vi "Translate Percent Codes.vi"(11 "String":string) -> (3 "String 2":string)   [LabVIEW 2019]
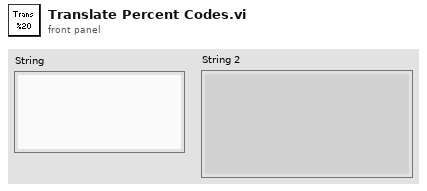
[diagram p1: front panel]
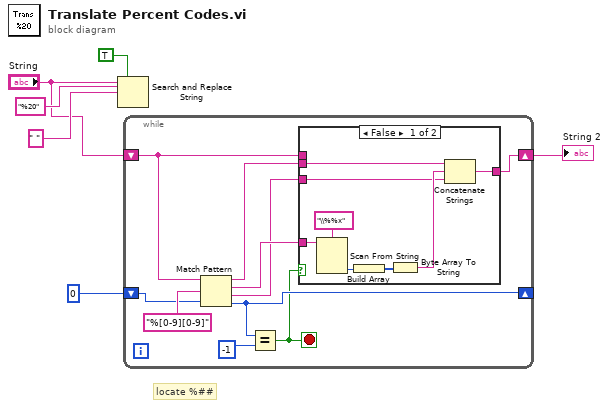
[diagram p0: block diagram]
diagram:
  # "locate %##"
  n1 = Search and Replace String(replace all?=TRUE ("replace all? (F)"), input string="String", search string="%20", replace string=" " ("search string")) -> ()  [unwired: 4 in, 4 out]
  n2 = while {
    shift-right: [w13] -> _
    shift-left: 0 ("offset past token") -> [w14]
    shift-right: [w10] -> w2
    shift-left: "String" -> [w8]
    stop <- w12 stop-if-true
    n3 = Match Pattern(string=w8, regular expression="%[0-9][0-9]" ("search string"), offset (0)=w14) -> (before substring=w11:string, match substring=w9:string, after substring=w7:string, offset past match=w13:i32)
    n4 = Equal?(x=w13, y=-1 ("offset past token")) -> (x = y?=w12:bool)
    n5 = case shown="False" w12 {
      tunnel: w11 -> [w24 _]
      tunnel: [w23 w25] -> w10
      tunnel: w8 -> [_ w25]
      tunnel: w9 -> [w22 _]
      tunnel: w7 -> [w17 _]
      frame False {
        n6 = Scan From String(format string="\\%%x" ("search string"), input string=w22) -> (output 1=w20:u32)  [unwired: 3 in, 3 out]
        n7 = Build Array(w20) -> (w19:u32[])
        n8 = Byte Array To String(unsigned byte array=w19) -> (string=w18:string)
        n9 = Concatenate Strings(w24, w18, w17) -> (w23:string)
      }
      frame True {
      }
    }
  }
  "String 2" <- w2
